vi "Set Color to cell.vi"(8 "error in (no error)":errorcluster, 9 "Active Cell:Active Cell":T1={"Row"=-2, "Column"=-2}, 10 "Color Box":u32(colorbox)=16448250, 11 "MCLB_Lib in":refnum<class "MCLB_Lib.lvclass">) -> (0 "error out":errorcluster, 3 "MCLB_Lib out":refnum<class "MCLB_Lib.lvclass">)   [LabVIEW 2020, in "MCLB_Lib.lvclass"]
uses:
  MCLB_Lib.lvclass
  <vilib>/Utility/miscctls.llb/LVRowAndColumnTypeDef.ctl
  MCLB_Lib.lvclass/MCLB_Lib.ctl
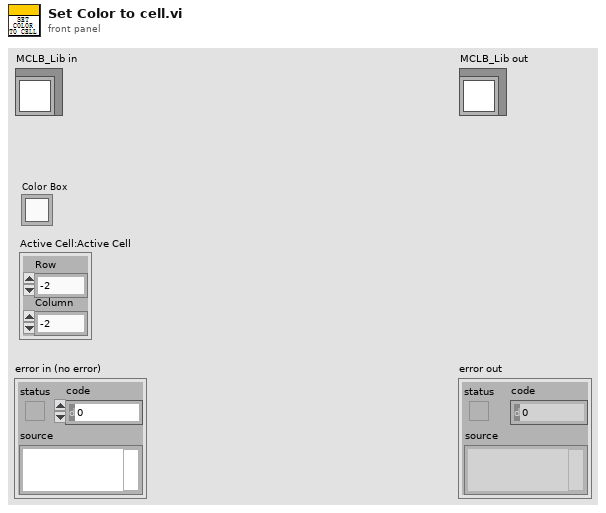
[diagram p1: front panel]
types:
  T1 = typedef "LVRowAndColumnTypeDef.ctl" = cluster{"Row":i32, "Column":i32}
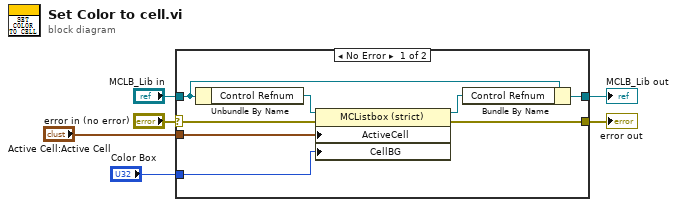
[diagram p0: block diagram]
diagram:
  n1 = case shown="No Error" "error in (no error)" {
    selector: "error in (no error)" -> [w10 w16]
    tunnel: [w9 w16] -> w3
    tunnel: [w12 w15] -> w5
    tunnel: "MCLB_Lib in" -> [w14 w15]
    tunnel: "Color Box" -> [w8 _]
    tunnel: "Active Cell:Active Cell" -> [w7 _]
    frame No Error {
      n2 = Unbundle By Name(w14) -> ("Control Refnum"=w13:refnum<vi>)
      n3 = property class="MCListbox (strict)"(reference=w13, error in=w10, "ActiveCell"=w7, "CellBG"=w8) -> (reference out=w11:refnum<vi>, error out=w9:errorcluster)
      n4 = Bundle By Name(cluster=w14, "Control Refnum"=w11) -> (w12:refnum<class "MCLB_Lib.lvclass">)
    }
    frame Error {
    }
  }
  "error out" <- w3
  "MCLB_Lib out" <- w5
